vi "umd_thermistor.vi"(8 "ready for output (T)":bool=TRUE, 9 "input valid":bool=TRUE, 10 "V":fxp<+/-,24,5>) -> (1 "ready for input":bool, 2 "Temperature":fxp<+/-,32,16>)   [LabVIEW 2018]
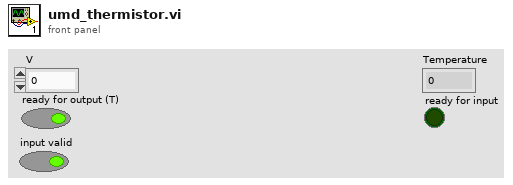
[diagram p1: front panel]
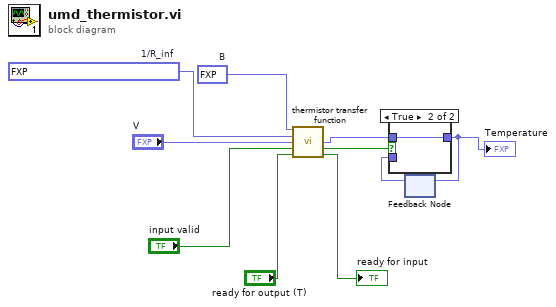
[diagram p0: block diagram]
diagram:
  w10 = fxp<+,32,7> 10.047783523797989  # 1/R_inf
  w9 = fxp<+/-,32,16> 3434.0  # B
  n1 = call "thermistor transfer function.vi"("B"=w9, "1/R_inf"=w10, "V"="V", "input valid"="input valid", "ready for output (T)"="ready for output (T)") -> ("Temperature"=w3:fxp<+/-,32,16>, "output valid"=w4:bool, "ready for input"=→"ready for input":bool)  [unwired: 8 in]
  n2 = feedback #1() -> (w1:fxp<+/-,32,16>)  [unwired: 1 in]
  n3 = case shown="True" w4 {
    tunnel: w3 -> [_ w12]
    tunnel: [w11 w12] -> w2
    tunnel: w1 -> [w11 _]
    frame False {
    }
    frame True {
    }
  }
  "Temperature" <- w2
  n4 = feedback-in #1(w2) -> ()
